vi "McLeodd method RT.vi"(8 "Next Amp":dbl, 9 "Max Amp":dbl, 10 "Max Bin":i32, 11 "Prev Amp":dbl) -> (2 "Bin":dbl)   [LabVIEW 2014]
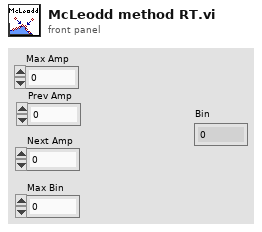
[diagram p1: front panel]
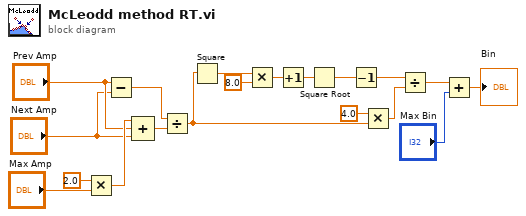
[diagram p0: block diagram]
diagram:
  n1 = Multiply(x=2.0, y="Max Amp") -> (x*y=w18:dbl)
  n2 = Subtract(x="Prev Amp", y="Next Amp") -> (x-y=w16:dbl)
  n3 = Compound Arithmetic op=ADD(w18, "Prev Amp", "Next Amp") -> (w17:dbl)
  n4 = Divide(x=w16, y=w17) -> (x/y=w9:dbl)
  n5 = Square(x=w9) -> (x^2=w15:dbl)
  n6 = Multiply(x=w15, y=8.0) -> (x*y=w13:dbl)
  n7 = Increment(x=w13) -> (x+1=w12:dbl)
  n8 = Square Root(x=w12) -> (sqrt(x)=w11:dbl)
  n9 = Decrement(x=w11) -> (x-1=w8:dbl)
  n10 = Multiply(x=4.0, y=w9) -> (x*y=w7:dbl)
  n11 = Divide(x=w8, y=w7) -> (x/y=w6:dbl)
  n12 = Add(x=w6, y="Max Bin") -> (x+y=→"Bin":dbl)
